vi "PicoScope2000WrapSetEnabledChannels.vi"(0 "Acquisition Settings":T1={"Auto Stop"=FALSE, "Desired Sample Interval"=2, "Max Samples"=333000, "Num Samples per Aggregate"=1, "Overview Buffer Size"=1000000, "Time Units"=3, "Application Buffer Size"=1500000} {"Application Buffer Size" format="%#_6p"; "Time Units" items=["Nanoseconds (ns)"=2, "Microseconds (us)"=3, "Milliseconds (ms)"=4, "Seconds (s)"=5]; "Overview Buffer Size" format="%#.5p"; "Max Samples" format="%#.5p"}, 4 "Channel B Settings":T2={"Enabled"=FALSE, "Coupling"=1, "Range"=6} {"Range" items=["20 mV"=1, "50 mV"=2, "100 mV"=3, "200 mV"=4, "500 mV"=5, "1 V"=6, "2 V"=7, "5 V"=8, "10 V"=9, "20 V"=10]; "Coupling" items=["AC", "DC"]}, 5 "Channel A Settings":T2={"Enabled"=FALSE, "Coupling"=1, "Range"=6} {"Range" items=["20 mV"=1, "50 mV"=2, "100 mV"=3, "200 mV"=4, "500 mV"=5, "1 V"=6, "2 V"=7, "5 V"=8, "10 V"=9, "20 V"=10]; "Coupling" items=["AC", "DC"]}, 6 "handle in":i16, 7 "error in (no error)":errorcluster) -> (2 "handle out":i16, 3 "error out":errorcluster)   [LabVIEW 2010]
uses:
  ps2000Wrap.dll
  PicoScope2000AnalogChannelSettings.ctl
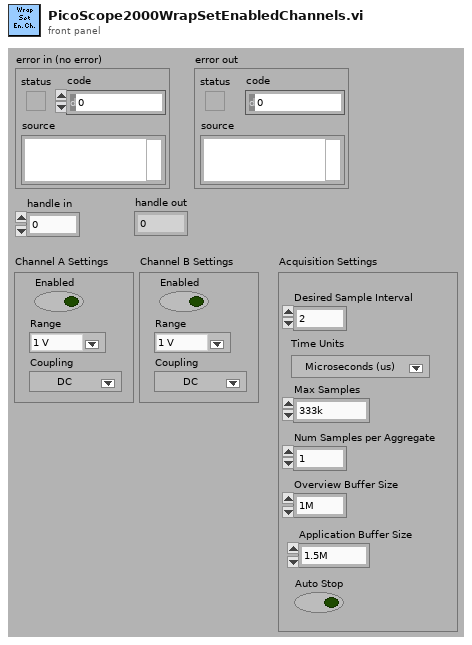
[diagram p1: front panel]
types:
  T1 = cluster{"Auto Stop":bool, "Desired Sample Interval":u32, "Max Samples":u32, "Num Samples per Aggregate":u32, "Overview Buffer Size":u32, "Time Units":u32, "Application Buffer Size":u32}
  T2 = typedef "PicoScope2000AnalogChannelSettings.ctl" = cluster{"Enabled":bool, "Coupling":i16, "Range":u16}
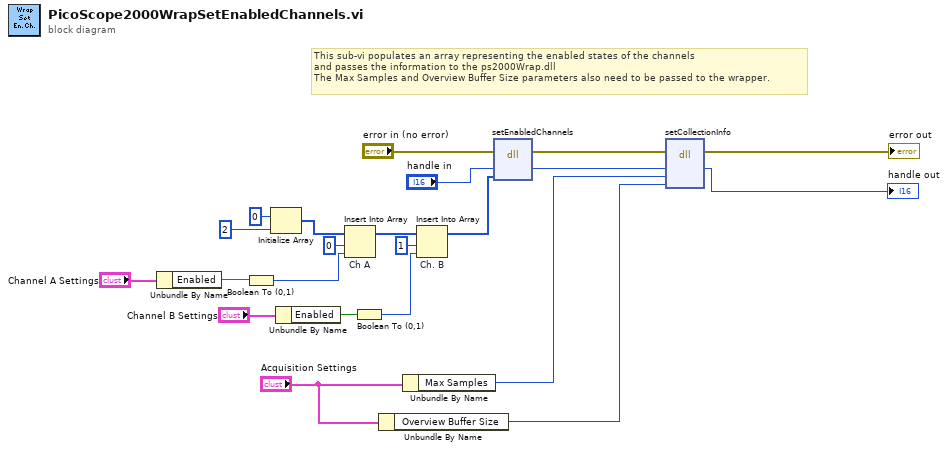
[diagram p0: block diagram]
diagram:
  # "This sub-vi populates an array representing the enabled states of the channels\nand passes the information to the ps2000Wrap.dll\nThe Max Samples and Overview Buffer Size parameters also need to be passed to the wrapper."
  n1 = Unbundle By Name("Channel A Settings") -> ("Enabled"=w12:bool)
  n2 = Boolean To (0,1)(Boolean=w12) -> (0, 1=w11:i16)
  n3 = Initialize Array "Initialize Array"(i16 0 ("element"), 2 ("dimension size")) -> (w19:i16[])
  n4 = Unbundle By Name("Channel B Settings") -> ("Enabled"=w10:bool)
  n5 = Insert Into Array "Ch A"(array=w19, index=0, new element=w11) -> (w18:i16[])
  n6 = Boolean To (0,1)(Boolean=w10) -> (0, 1=w9:i16)
  n7 = Unbundle By Name("Acquisition Settings") -> ("Overview Buffer Size"=w1:u32)
  n8 = Unbundle By Name("Acquisition Settings") -> ("Max Samples"=w3:u32)
  n9 = Insert Into Array "Ch. B"(array=w18, index=1, new element=w9) -> (w15:i16[])
  n10 = dll-call lib="ps2000Wrap.dll" fn="setEnabledChannels"(error in="error in (no error)", "handle"="handle in", "enabledChannels"=w15) -> (error out=w6:errorcluster, "handle"=w8:i16)  [unwired: 4 in, 1 out]
  n11 = dll-call lib="ps2000Wrap.dll" fn="setCollectionInfo"(error in=w6, "handle"=w8, "collectionSize"=w3, "overviewBufferSize"=w1) -> (error out=→"error out":errorcluster, "handle"=→"handle out":i16)  [unwired: 5 in, 1 out]
